vi "constants_FPGA.vi"(8 "error in (no error)":errorcluster) -> (0 "error out":errorcluster, 1 "batch updater file path":path, 2 "file path for Signal .hdf5 files":path, 3 "DB connection File Path":path, 4 "file path for Processed Signal .hdf5 files":path, 5 "Testing":bool=TRUE, 6 "Private Folder file path":path)   [LabVIEW 2012]
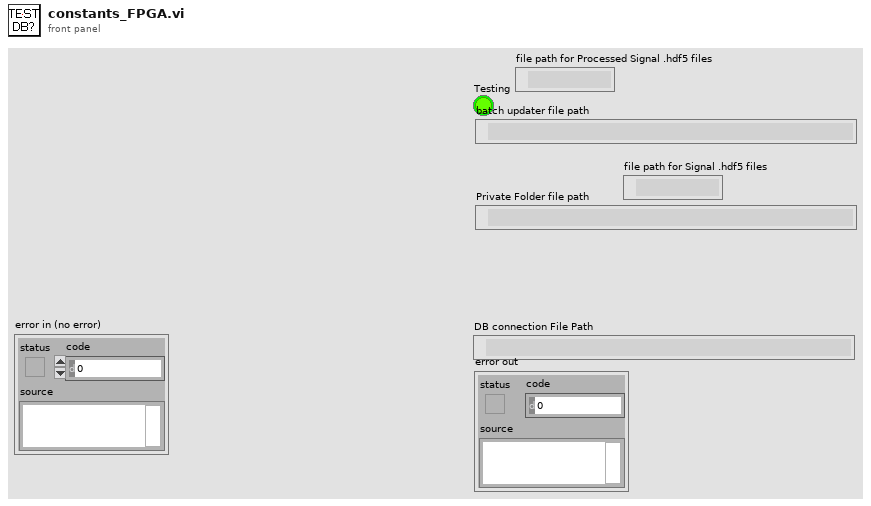
[diagram p1: front panel]
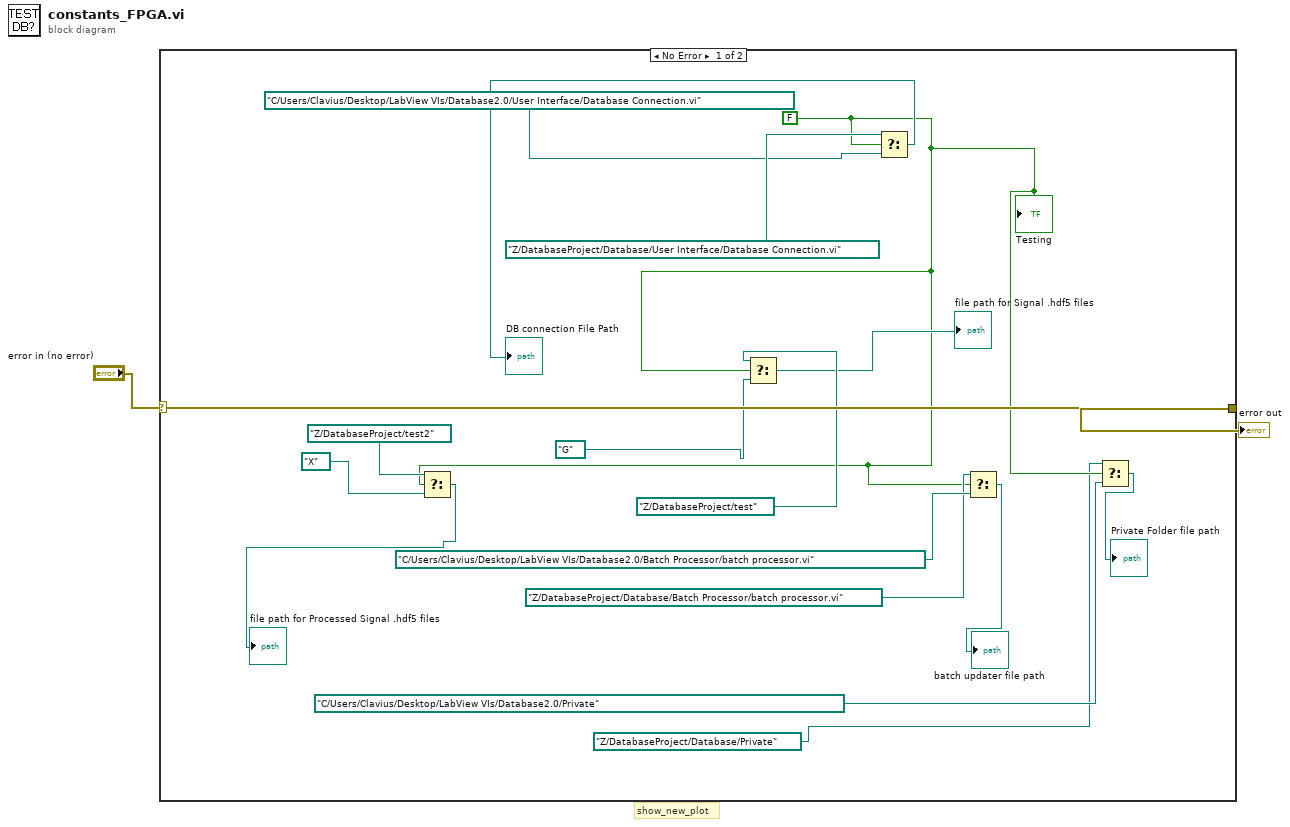
[diagram p0: block diagram]
diagram:
  # "show_new_plot"
  n1 = case shown="No Error" "error in (no error)" {
    selector: "error in (no error)" -> [w16 w20]
    tunnel: [w16 w20] -> w2
    frame No Error {
      w6 = FALSE ("Testing")
      n2 = Select(t=path "Z:/DatabaseProject/test2", s=w6, f=path "X:/") -> (s? t:f=→"file path for Processed Signal .hdf5 files":path)
      n3 = Select(t=path "Z:/DatabaseProject/test", s=w6, f=path "G:/") -> (s? t:f=→"file path for Signal .hdf5 files":path)
      n4 = Select(t=path "Z:/DatabaseProject/Database/User Interface/Database Connection.vi", s=w6, f=path "C:/Users/Clavius/Desktop/LabView VIs/Database2.0/User Interface/Database Connection.vi" ("vi path")) -> (s? t:f=→"DB connection File Path":path)
      n5 = Select(t=path "Z:/DatabaseProject/Database/Batch Processor/batch processor.vi", s=w6, f=path "C:/Users/Clavius/Desktop/LabView VIs/Database2.0/Batch Processor/batch processor.vi" ("vi path")) -> (s? t:f=→"batch updater file path":path)
      n6 = Select(t=path "Z:/DatabaseProject/Database/Private", s=w6, f=path "C:/Users/Clavius/Desktop/LabView VIs/Database2.0/Private" ("vi path")) -> (s? t:f=→"Private Folder file path":path)
      "Testing" <- w6
    }
    frame Error {
    }
  }
  "error out" <- w2
